vi "First_Touch_Fisher.vi"() -> ()   [LabVIEW 2013]
uses:
  Instance           1 22Saved   HandsOn onkija .vi
panel:
  in  "Bottom amplitude":dbl=1.0 caption="Amplitude"
  in  "Wave frequency\nstart value 0,001":dbl=10.1 caption="Frequency"
  in  "Bottom frequency (Hz)\nMeaningfull a.0,0001":dbl=0.1 caption="Frequency"
  in  "Bottom offset":dbl=1.0 caption="Amplitude"
  in  "Wave amplitude \nstart value 0,1":dbl=1.0 caption="Amplitude"
  out "Lake waves":dynamicdata(graph)
  in  "stop":bool
  in  "Line length (control)":dbl(slide) scale=0.0..10.0
  out "RED bottom\nGreen OK":bool
  out "line length (indicator)":dbl(knob) scale=0.0..10.0
  out "Lake bottom":dynamicdata(graph)
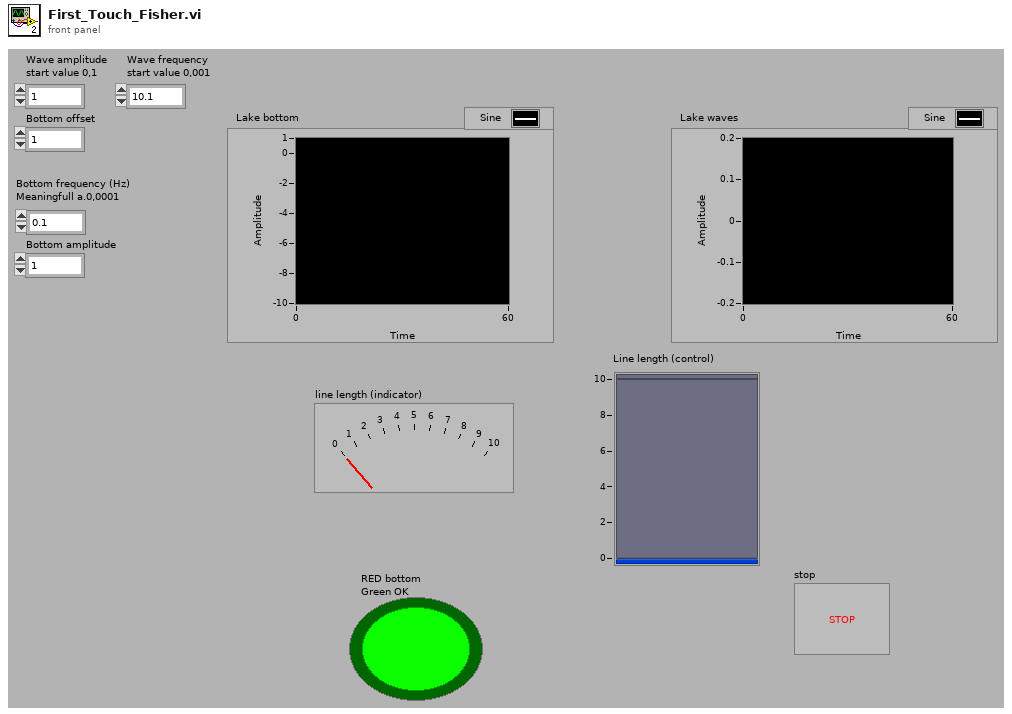
[diagram p1: front panel]
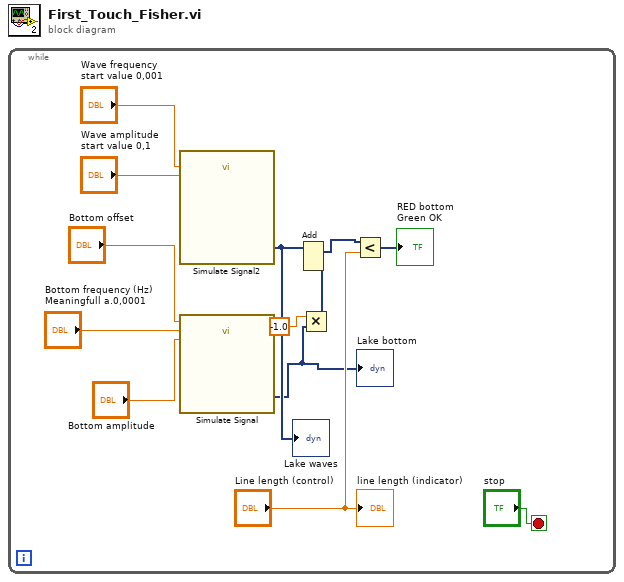
[diagram p0: block diagram]
diagram:
  n1 = while {
    stop <- "stop" stop-if-true
    n2 = call "Simulate Signal2"("Frequency"="Wave frequency\nstart value 0,001", "Amplitude"="Wave amplitude \nstart value 0,1") -> ("Sine"=w11:dynamicdata)  [unwired: 12 in, 1 out]
    "Lake waves" <- w11
    n3 = call "Simulate Signal"("Offset"="Bottom offset", "Frequency"="Bottom frequency (Hz)\nMeaningfull a.0,0001", "Amplitude"="Bottom amplitude") -> ("Sine"=w1:dynamicdata)  [unwired: 11 in, 1 out]
    "Lake bottom" <- w1
    n4 = Multiply(x=-1.0, y=w1) -> (x*y=w3:dynamicdata)
    n5 = Add(1:w3, 2:w11) -> (0:w5:dynamicdata)  [unwired: 1 in, 1 out]
    n6 = Less?(x=w5, y="Line length (control)") -> (x < y?=→"RED bottom\nGreen OK":dynamicdata)
    "line length (indicator)" <- "Line length (control)"
  }
